vi "Refactor Dependencies for Projects.vi"() -> ()   [LabVIEW 2021, in "MeasurementService Editor.lvlib"]
uses:
  MeasurementService Editor.lvlib
  Refactor Object Result.ctl
  Refactor Dynamic Dispatch Member Result.ctl
  Refactor Project Result.ctl
  Rename String.ctl
  Rename String Result.ctl
panel:
  in  "Refactor Data":u16(ring)=1 items=["V1 to V2 (Jan 2024)", "V2 to V3 (July 2024)"]
  out "refactor results":T1[](array[typedef])
  out "projects with errors":i32
  out "status string":string
  in  "stop":bool
  in  "project file or folder (recursive)":path
  # "These refactorings are not cumulative. If you have code from before the refactor date, run them in series starting with the oldest one."
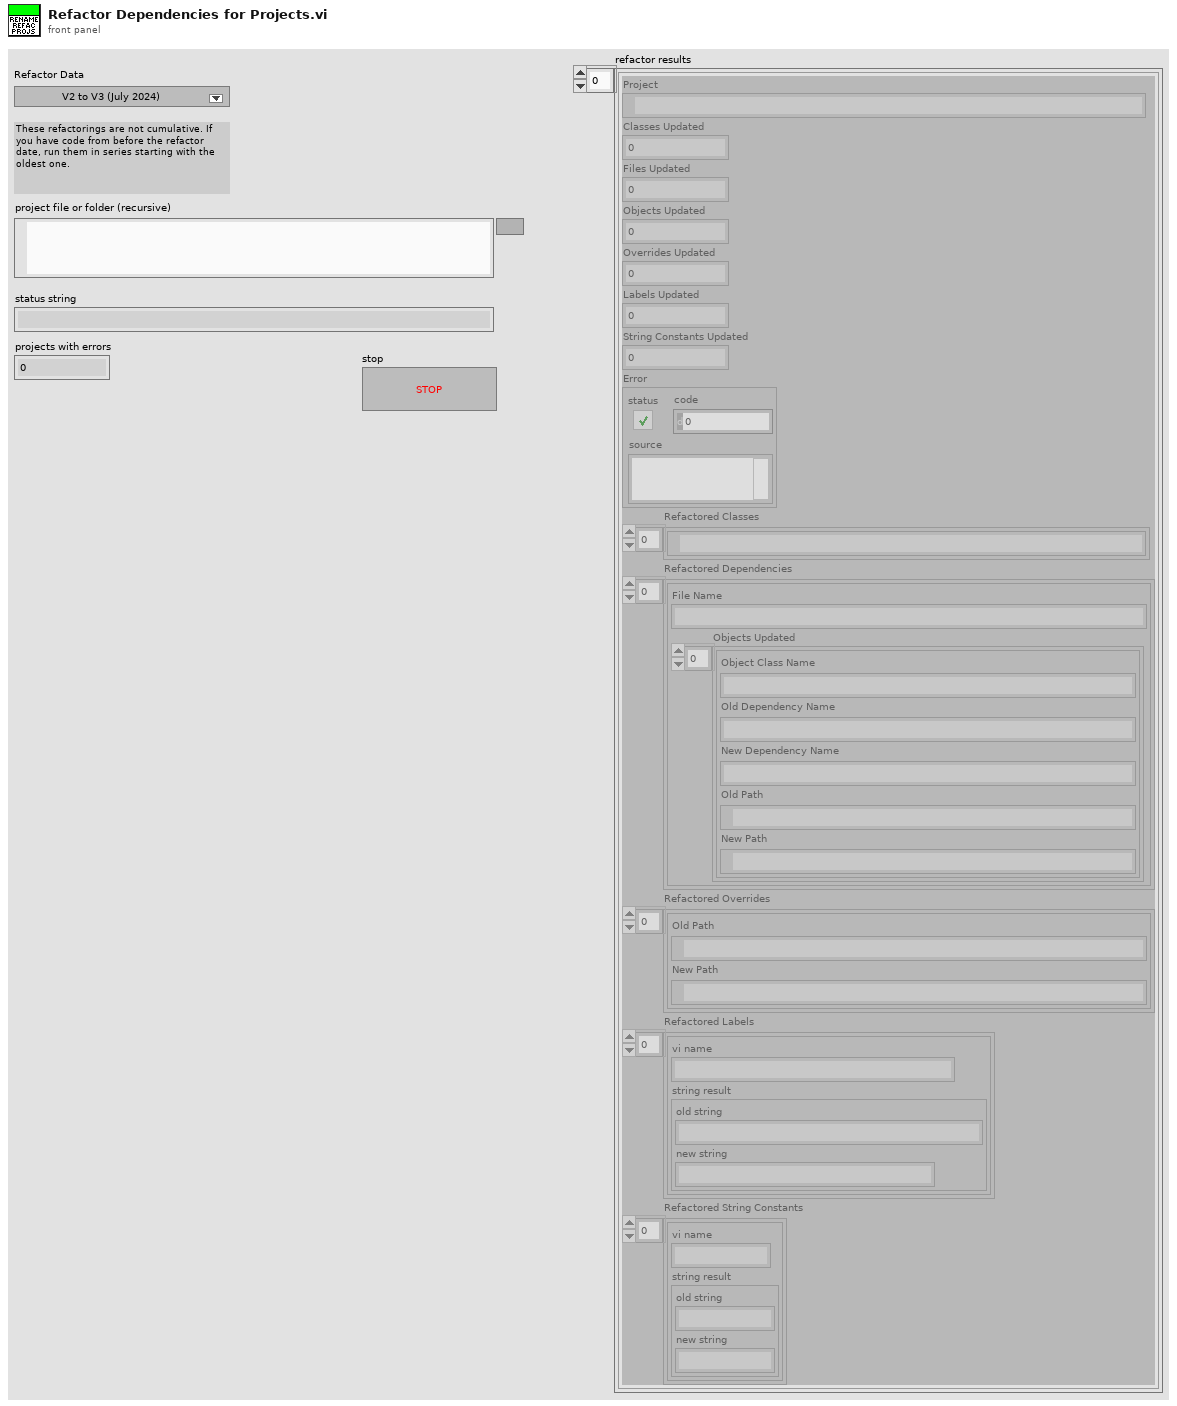
[diagram p1: front panel]
types:
  T1 = typedef "MeasurementService Editor.lvlib/Refactor Project Result.ctl" = cluster{"Project":path, "Classes Updated":u32, "Files Updated":u32, "Objects Updated":u32, "Overrides Updated":u32, "Labels Updated":u32, "String Constants Updated":u32, "Error":errorcluster, "Refactored Classes":path[], "Refactored Dependencies":cluster{"File Name":string, "Objects Updated":T2[]}[], "Refactored Overrides":T3[], "Refactored Labels":T4[], "Refactored String Constants":T4[]}
  T2 = typedef "MeasurementService Editor.lvlib/Refactor Object Result.ctl" = cluster{"Object Class Name":string, "Old Dependency Name":string, "New Dependency Name":string, "Old Path":path, "New Path":path}
  T3 = typedef "MeasurementService Editor.lvlib/Refactor Dynamic Dispatch Member Result.ctl" = cluster{"Old Path":path, "New Path":path}
  T4 = typedef "MeasurementService Editor.lvlib/Rename String Result.ctl" = cluster{"vi name":string, "string result":T5}
  T5 = typedef "MeasurementService Editor.lvlib/Rename String.ctl" = cluster{"old string":string, "new string":string}
  T6 = typedef "Copy of MeasurementService Editor.lvlib/Rename Refactor Data.ctl" = cluster{"Renamed Libraries":T7[], "Renamed Files":T7[], "Dynamic to Static Dispatch Members":T7[], "Renamed Control Labels":T8[], "Renamed String Constants":T8[]}
  T7 = typedef "Copy of MeasurementService Editor.lvlib/Rename Refactor Mapping Info.ctl" = cluster{"Old Name":string, "Old Directory":path, "New Name":string, "New Directory":path}
  T8 = typedef "Copy of MeasurementService Editor.lvlib/Rename String Mapping.ctl" = cluster{"vi name":string, "old string":string[], "new string":string[]}
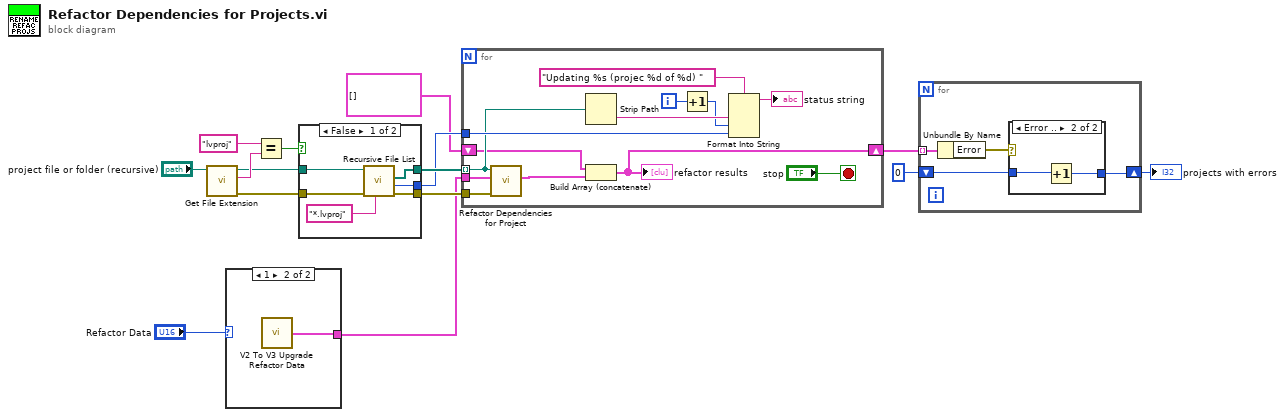
[diagram p0: block diagram]
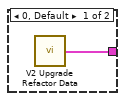
[diagram p2: hidden frame]
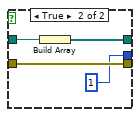
[diagram p3: hidden frame]
diagram:
  n1 = call <vilib>:"Get File Extension.vi"("file"="project file or folder (recursive)") -> ("error out"=w7:errorcluster, "lowercase file extension"=w6:string, "dup file"=w3:path)  [unwired: 6 in, 2 out]
  n2 = case shown="1" "Refactor Data" {
    tunnel: [w16 w17] -> w1
    frame 0, Default {
      n3 = call "V2 Upgrade Refactor Data.vi"() -> ("refactor data"=w16:T6)
    }
    frame 1 {
      n4 = call "V2 To V3 Upgrade Refactor Data.vi"() -> ("refactor data"=w17:T6)
    }
  }
  n5 = Equal?(x="lvproj", y=w6) -> (x = y?=w4:bool)
  n6 = case shown="False" w4 {
    tunnel: [w22 w25] -> w15
    tunnel: [w21 w26] -> w14
    tunnel: [w20 1 ("Number of Files")] -> w13
    tunnel: w7 -> [w19 w26]
    tunnel: w3 -> [w18 w27]
    frame False {
      n7 = call <vilib>:"Recursive File List.vi"("pattern"="*.lvproj", "error in (no error)"=w19, "Folder Path"=w18) -> ("error out"=w21:errorcluster, "Number of Files"=w20:i32, "All Files in Dir"=w22:path[])  [unwired: 4 in, 2 out]
    }
    frame True {
      n8 = Build Array(w27) -> (w25:path[])
    }
  }
  n9 = for {
    tunnel: w15 -> [w31] mode=indexing
    tunnel: w1 -> [w40]
    tunnel: w14 -> [w39]
    tunnel: w13 -> [w33]
    shift-right: [w28] -> w11
    shift-left: T1[] [] ("refactor results") -> [w30]
    i -> [w37]
    stop <- "stop" stop-if-true
    n10 = call "Refactor Dependencies for Project.vi"("error in (no error)"=w39, "refactor data"=w40, "project path"=w31) -> ("refactor result"=w29:T1)  [unwired: 7 in, 1 out]
    n11 = Strip Path(path=w31) -> (name=w35:string)  [unwired: 1 out]
    n12 = Build Array (concatenate)(w30, w29) -> (w28:T1[])
    "refactor results" <- w28
    n13 = Increment(x=w37) -> (x+1=w34:i32)
    n14 = Format Into String(format string="Updating %s (projec %d of %d) ", w35, w34, w33) -> (resulting string=→"status string":string)  [unwired: 2 in, 1 out]
  }
  n15 = for {
    tunnel: w11 -> [w44] mode=indexing
    shift-right: [w41] -> w9
    shift-left: 0 ("x") -> [w42]
    n16 = Unbundle By Name(w44) -> ("Error"=w43:errorcluster)
    n17 = case shown="Error .." w43 {
      tunnel: w42 -> [w45 w47]
      tunnel: [w45 w46] -> w41
      frame No Error {
      }
      frame Error {
        n18 = Increment(x=w47) -> (x+1=w46:i32)
      }
    }
  }
  "projects with errors" <- w9
